vi "nesnetespiti.vi"() -> ()   [LabVIEW 2017]
panel:
  in  "Search Rect (entire image)":T1 {"Rotation" format="%.2f"; "Left" scale=0.0..1024.0; "Right" scale=0.0..1024.0}
  out "Number of Objects":i32
  out "error out":errorcluster
  in  "Settings":T2={"Objects"=0, "Threshold"=128, "Reject Border"=FALSE, "Fill Holes"=FALSE, "Min Object Size"=FALSE, "Min Size"=3, "Max Object Size"=FALSE, "Max Size"=100, "Show Search Area"=FALSE, "Show Center"=TRUE, "Show Bounding Box"=TRUE} {"Objects" items=["Bright Objects", "Dark Objects"]; "Threshold" min=1 max=999999999 step=1; "Max Size" min=1 max=999999999 step=1; "Min Size" min=1 max=999999999 step=1}
  in  "File Path":path
  out "Image":T3(plugin-control)
  in  "Image Type":T4 items=["Grayscale (U8)", "Grayscale (I16)", "Grayscale (SGL)", "Complex (CSG)", "RGB (U32)", "HSL (U32)", "RGB (U64)", "Grayscale (U16)"]
  in  "stop":bool
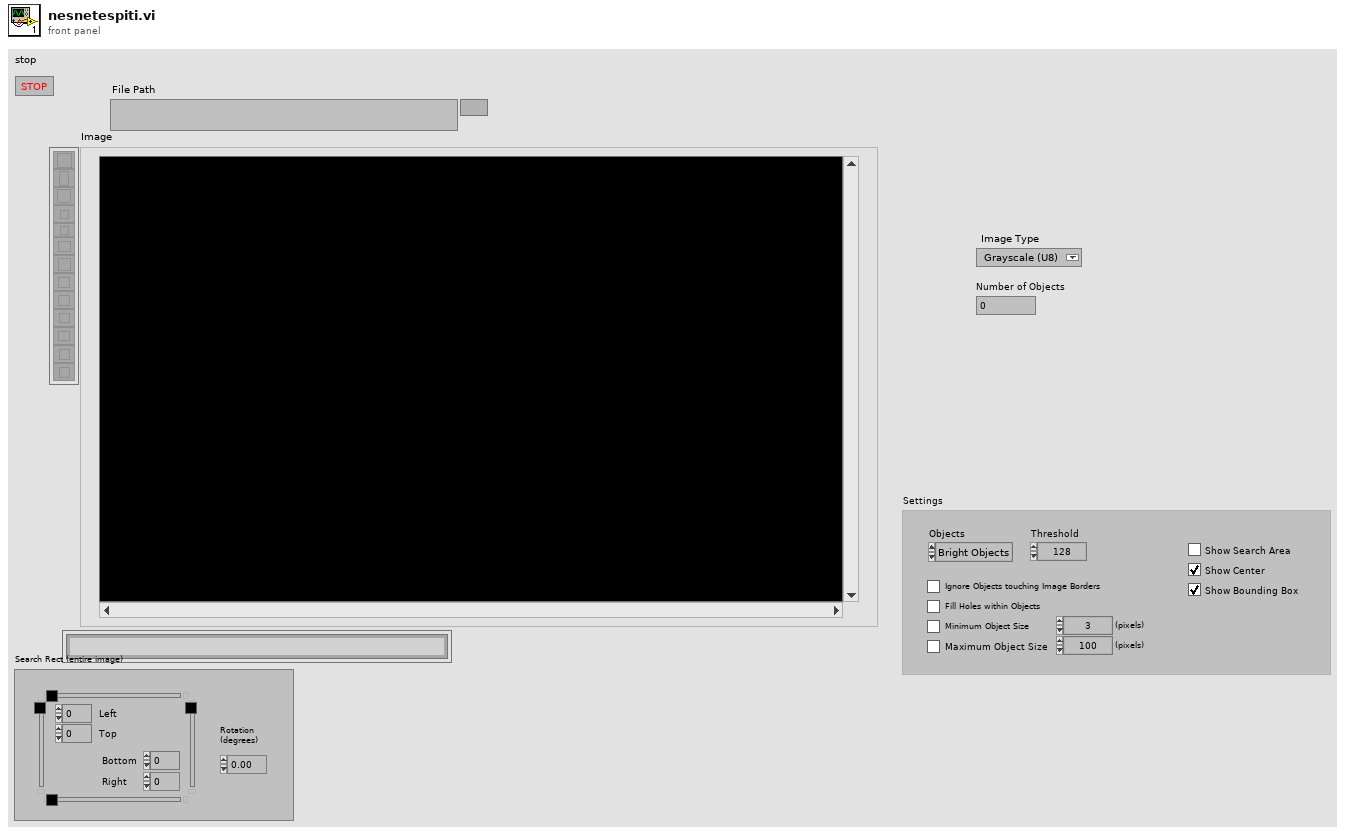
[diagram p1: front panel]
types:
  T1 = typedef "IMAQ Rectangle" = cluster{"Left":i32, "Top":i32, "Right":i32, "Bottom":i32, "Rotation":dbl}
  T2 = cluster{"Objects":u16, "Threshold":i32, "Reject Border":bool, "Fill Holes":bool, "Min Object Size":bool, "Min Size":i32, "Max Object Size":bool, "Max Size":i32, "Show Search Area":bool, "Show Center":bool, "Show Bounding Box":bool}
  T3 = typedef "IMAQ Image.ctl" = refnum<image>
  T4 = typedef "Image Type" = u32
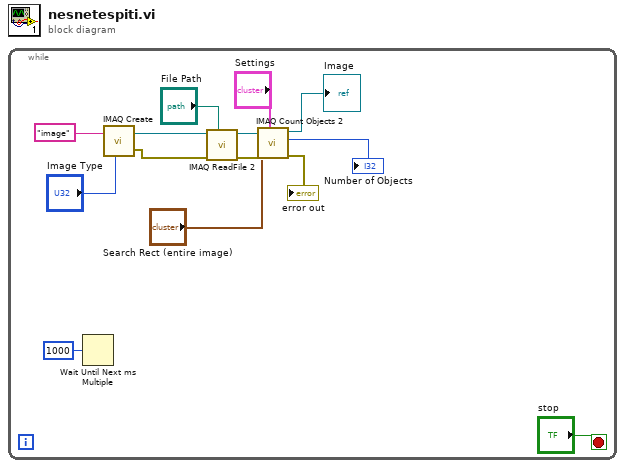
[diagram p0: block diagram]
diagram:
  n1 = while {
    stop <- "stop" stop-if-true
    n2 = Wait Until Next ms Multiple(millisecond multiple=u32 1000) -> ()  [unwired: 1 out]
    n3 = call "IMAQ Create"("Image Name"="image", "Image Type"="Image Type") -> ("New Image"=w11:T3, "error out"=w5:errorcluster)  [unwired: 3 in]
    n4 = call "IMAQ ReadFile 2"("File Path"="File Path", "error in (no error)"=w5, "Image"=w11) -> ("error out"=w4:errorcluster, "Image Out"=w10:T3)  [unwired: 4 in, 3 out]
    n5 = call "IMAQ Count Objects 2"("Settings"="Settings", "error in (no error)"=w4, "Search Rect (entire image)"="Search Rect (entire image)", "Image"=w10) -> ("error out"=→"error out":errorcluster, "Number of Objects"=→"Number of Objects":i32, "Image Out"=→"Image":T3)  [unwired: 3 in, 2 out]
  }
